vi "Read_IR.vi"(0 "error in":errorcluster, 2 "Side":T2, 3 "node":string) -> (1 "error out":errorcluster, 4 "Range Data":T1)   [LabVIEW 2012]
doc: "Read the IR (either right or left)."
uses:
  <userlib>/ROSforLV/ROS/Code/SubVIs/BaxterSide.ctl
  <userlib>/ROSforLV/ROS/Code/Console/Servers/ServerSubs/TopicDef.ctl
  <userlib>/ROSforLV/ROS/Code/SubVIs/_ROSDirection.ctl
panel:
  out "Reply":string
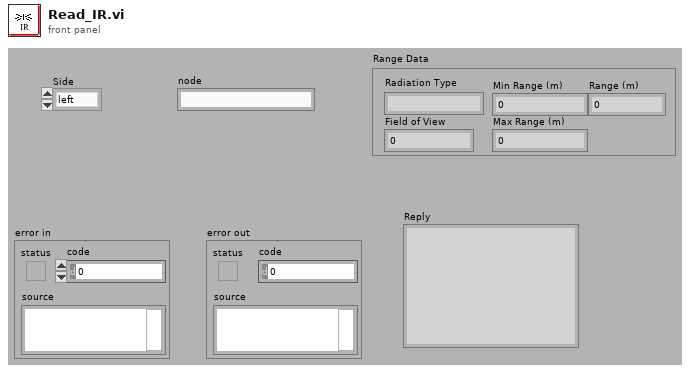
[diagram p1: front panel]
types:
  T1 = cluster{"Radiation Type":string, "Field of View":sgl, "Min Range (m)":sgl, "Max Range (m)":sgl, "Range (m)":sgl}
  T2 = typedef "BaxterSide.ctl" = enum16{"left", "right"}
  T3 = typedef "TopicDef.ctl" = cluster{"Topic":string, "Type":string, "Action":T4, "Update (ms)":u16, "queue size":u16}
  T4 = typedef "_ROSDirection.ctl" = enum16{"Node", "Publisher", "Subscriber", "Service Client"}
  T5 = typedef "_ROSControl.ctl" = cluster{"topic port":u16, "Node":string, "topic":string, "type":string, "node port":u16, "error ":errorcluster, "Direction":T4, "Update (ms)":u16, "queue size":u16}
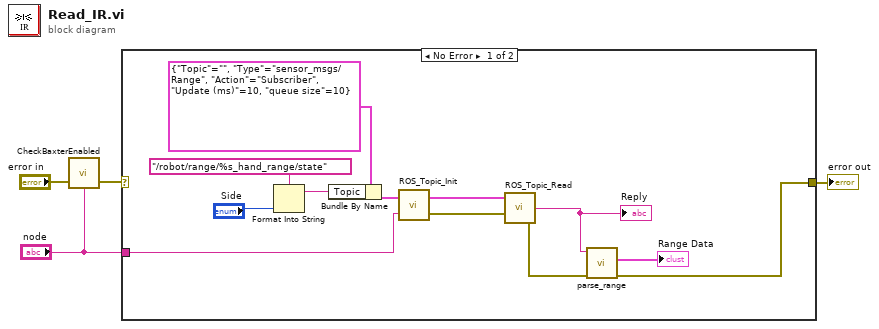
[diagram p0: block diagram]
diagram:
  n1 = call <userlib>:"CheckBaxterEnabled.vi"("error in"="error in", "node"="node") -> ("error out"=w2:errorcluster)  [unwired: 2 in]
  n2 = case shown="No Error" w2 {
    selector: w2 -> [_ w17]
    tunnel: [w5 w17] -> w4
    tunnel: "node" -> [w8 _]
    frame No Error {
      n3 = Format Into String(format string="/robot/range/%s_hand_range/state" ("topic"), "Side") -> (resulting string=w11:string)  [unwired: 2 in, 1 out]
      n4 = Bundle By Name(cluster=T3 {"Topic"="", "Type"="sensor_msgs/Range", "Action"=enum."Subscriber", "Update (ms)"=10, "queue size"=10} ("Definitions"), "Topic"=w11) -> (w9:T3)
      n5 = call <userlib>:"ROS_Topic_Init.vi"("node"=w8, "Definitions"=w9) -> ("error out"=w6:errorcluster, "ROS out"=w16:T5)
      n6 = call <userlib>:"ROS_Topic_Read.vi"("error in (no error)"=w6, "ROS in"=w16) -> ("error out"=w7:errorcluster, "Reply"=w14:string)  [unwired: 1 in, 1 out]
      "Reply" <- w14
      n7 = call <userlib>:"parse_range.vi"("error in"=w7, "msg in"=w14) -> ("error out"=w5:errorcluster, "Range Data"=→"Range Data":T1)  [unwired: 2 in, 2 out]
    }
    frame Error {
    }
  }
  "error out" <- w4
